vi "Configure Trigger (Pattern).vi"(0 "VISA resource name":refnum<visa-resource-name>, 1 "Minimum Time (20e-9s)":dbl=2e-08, 5 "Trigger Source (1: Channel1)":i32(ring)=1 items=["Channel1"=1, "Channel2"=2, "Channel3"=3, "Channel4"=4, "DIG0"=20, "DIG1"=21, "DIG2"=22, "DIG3"=23, "DIG4"=24, "DIG5"=25, "DIG6"=26, "DIG7"=27, "DIG8"=28, "DIG9"=29, "DIG10"=30, "DIG11"=31, "DIG12"=32, "DIG13"=33, "DIG14"=34, "DIG15"=35], 7 "Logic Criteria (0:High)":u16(ring) items=["High", "Low", "Don't Care", "Rising", "Falling"], 9 "Pattern Condition (0:Entered)":u16(ring) items=["Entered", "Exited", "Greater Than", "Less Than", "Range"], 11 "error in (no error)":errorcluster, 12 "Maximum Time (50e-9s)":dbl=5e-08) -> (4 "VISA resource name out":refnum<visa-resource-name>, 15 "error out":errorcluster)   [LabVIEW 2013, in "Agilent 90000 Series.lvlib"]
doc: "Configures the pattern trigger parameters."
uses:
  Agilent 90000 Series.lvlib
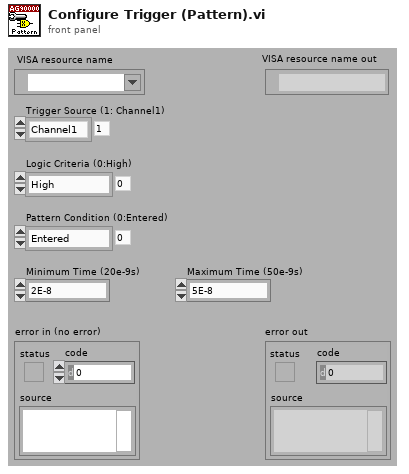
[diagram p1: front panel]
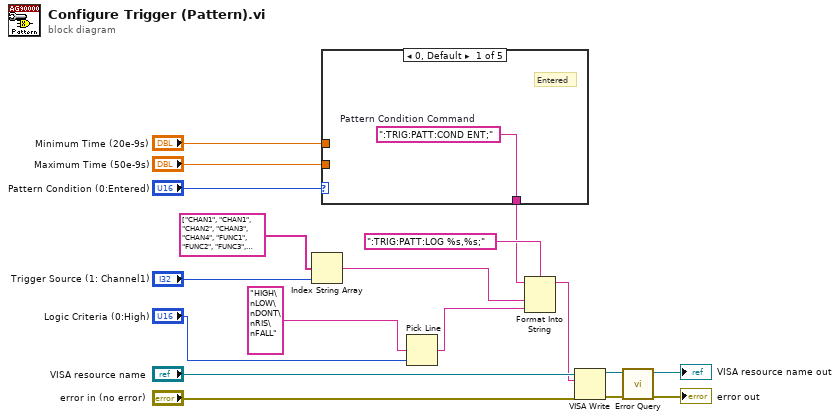
[diagram p0: block diagram]
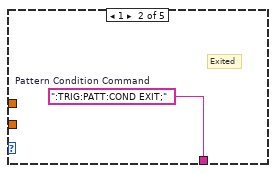
[diagram p2: hidden frame]
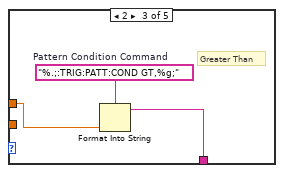
[diagram p3: hidden frame]
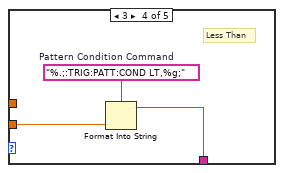
[diagram p4: hidden frame]
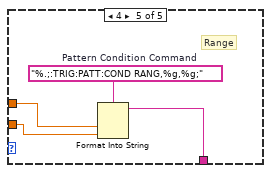
[diagram p5: hidden frame]
diagram:
  n1 = Index String Array(1:"Trigger Source (1: Channel1)", 2:string[] ["CHAN1", "CHAN1", "CHAN2", "CHAN3", "CHAN4", "FUNC1", "FUNC2", "FUNC3", "FUNC4", "WMEM1", "WMEM2", "WMEM3", "WMEM4", "AUX", "LINE", "", "", "", "", "", "DIG0", "DIG1", "DIG2", "DIG3", "DIG4", "DIG5", "DIG6", "DIG7", "DIG8", "DIG9", "DIG10", "DIG11", "DIG12", "DIG13", "DIG14", "DIG15", "", ""]) -> (0:w6:string)  [unwired: 1 out]
  n2 = case shown="0, Default" "Pattern Condition (0:Entered)" {
    tunnel: "Minimum Time (20e-9s)" -> [_ _ w22 _ w29]
    tunnel: "Maximum Time (50e-9s)" -> [_ _ _ w25 w28]
    tunnel: [w19 w20 w21 w24 w27] -> w4
    frame 0, Default {
      w19 = ":TRIG:PATT:COND ENT;"  # Pattern Condition Command
      # "Entered"
    }
    frame 1 {
      w20 = ":TRIG:PATT:COND EXIT;"  # Pattern Condition Command
      # "Exited"
    }
    frame 2 {
      w23 = "%.;:TRIG:PATT:COND GT,%g;"  # Pattern Condition Command
      # "Greater Than"
      n3 = Format Into String(format string=w23, w22) -> (resulting string=w21:string)  [unwired: 2 in, 1 out]
    }
    frame 3 {
      w26 = "%.;:TRIG:PATT:COND LT,%g;"  # Pattern Condition Command
      # "Less Than"
      n4 = Format Into String(format string=w26, w25) -> (resulting string=w24:string)  [unwired: 2 in, 1 out]
    }
    frame 4 {
      w30 = "%.;:TRIG:PATT:COND RANG,%g,%g;"  # Pattern Condition Command
      # "Range"
      n5 = Format Into String(format string=w30, w29, w28) -> (resulting string=w27:string)  [unwired: 2 in, 1 out]
    }
  }
  n6 = Pick Line(multi-line string="HIGH\nLOW\nDONT\nRIS\nFALL", line index="Logic Criteria (0:High)") -> (output string=w5:string)  [unwired: 1 out]
  n7 = Format Into String(format string=":TRIG:PATT:LOG %s,%s;", initial string=w4, w6, w5) -> (resulting string=w3:string)  [unwired: 1 in, 1 out]
  n8 = VISA Write(VISA resource name="VISA resource name", write buffer=w3, error in (no error)="error in (no error)") -> (VISA resource name out=w16:refnum<visa-resource-name>, error out=w15:errorcluster)  [unwired: 1 out]
  n9 = call "Error Query.vi"("error in (no error)"=w15, "VISA resource name"=w16) -> ("error out"=→"error out":errorcluster, "VISA resource name out"=→"VISA resource name out":refnum<visa-resource-name>)  [unwired: 8 out]
